vi "Example.vi"() -> ()   [LabVIEW 2024]
uses:
  LogHandle/Event/EventLogHandle.lvclass/EventLogHandle.ctl
  Record/LogRecord.lvclass/LogRecord.ctl
  Record/Read Message.vi
  Record/Read Source.vi
  LogHandle/Event/EventLogHandle.lvclass
  C:/Github/JQMH/JQMHCore/ErrorReporting/LoggingHandle/LoggingHandle.lvclass
  Record/LogRecord.lvclass
  RQMHLogger/RQMHLogger.lvclass
  HandleHolder/HandleHolder.lvclass
panel:
  out "Source":string
  out "Message":string
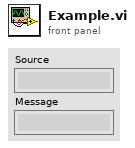
[diagram p1: front panel]
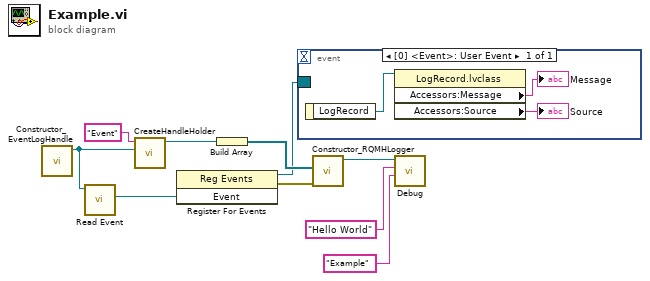
[diagram p0: block diagram]
diagram:
  n1 = call "Constructor_EventLogHandle.vi"() -> ("EventHandle"=w7:refnum<class "EventLogHandle.lvclass">)  [unwired: 10 in, 1 out]
  n2 = call "Read Event.vi"("EventLogHandle in"=w7) -> ("Event"=w6:refnum<user-event>)  [unwired: 8 in, 2 out]
  n3 = call "CreateHandleHolder.vi"("Handle"=w7, "Name"="Event") -> ("HandleHolder out"=w9:refnum<class "HandleHolder.lvclass">)  [unwired: 9 in]
  n4 = register-events(w6) -> (reference out=w5:refnum<event-registration>, error out=w1:errorcluster)  [unwired: 2 in]
  n5 = Build Array(w9) -> (w8:refnum<class "HandleHolder.lvclass">[])
  n6 = event shown="[0] <Event>: User Event" {
    selector: w5 -> [_]
    dyn-events: _ -> [_]
    timeout: _ -> [_]
    event User Event {
      n7 = event-data() -> ("LogRecord"=w13:refnum<class "LogRecord.lvclass">)  [unwired: 1 in]
      n8 = property class="LogRecord.lvclass"(reference=w13) -> ("Accessors:Message"=→"Message":string, "Accessors:Source"=→"Source":string)  [unwired: 1 in, 2 out]
    }
  }
  n9 = call "Constructor_RQMHLogger.vi"("error in (no error)"=w1, "Handles"=w8) -> ("RQMHLogger out"=w4:refnum<class "RQMHLogger.lvclass">)  [unwired: 8 in, 1 out]
  n10 = call "Debug.vi"("Source"="Example", "Message"="Hello World", "RQMHLogger in"=w4) -> ()  [unwired: 7 in, 2 out]
